vi "getData.vi"() -> (1 "Analogue Data (volts)":dbl[][](array[numeric]), 2 "Error Status":bool)   [LabVIEW 2017]
uses:
  Controls/blockTiming.ctl
  Globals/measurementGlobal.vi
panel:
  in  "display write dialog?":bool
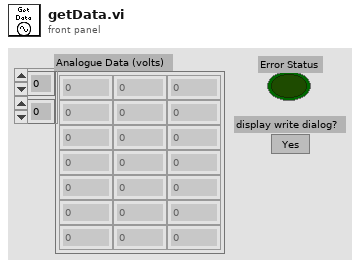
[diagram p1: front panel]
types:
  T1 = enum16{"New Measurement", "Post-process Raw Data"}
  T2 = typedef "blockTiming.ctl" = cluster{"Started":string, "Ended":string, "Analogue Frequency (Hz)":dbl}
  T3 = typedef "saveDataOption.ctl" = enum16{"Save Data", "Do Not Save Data"}
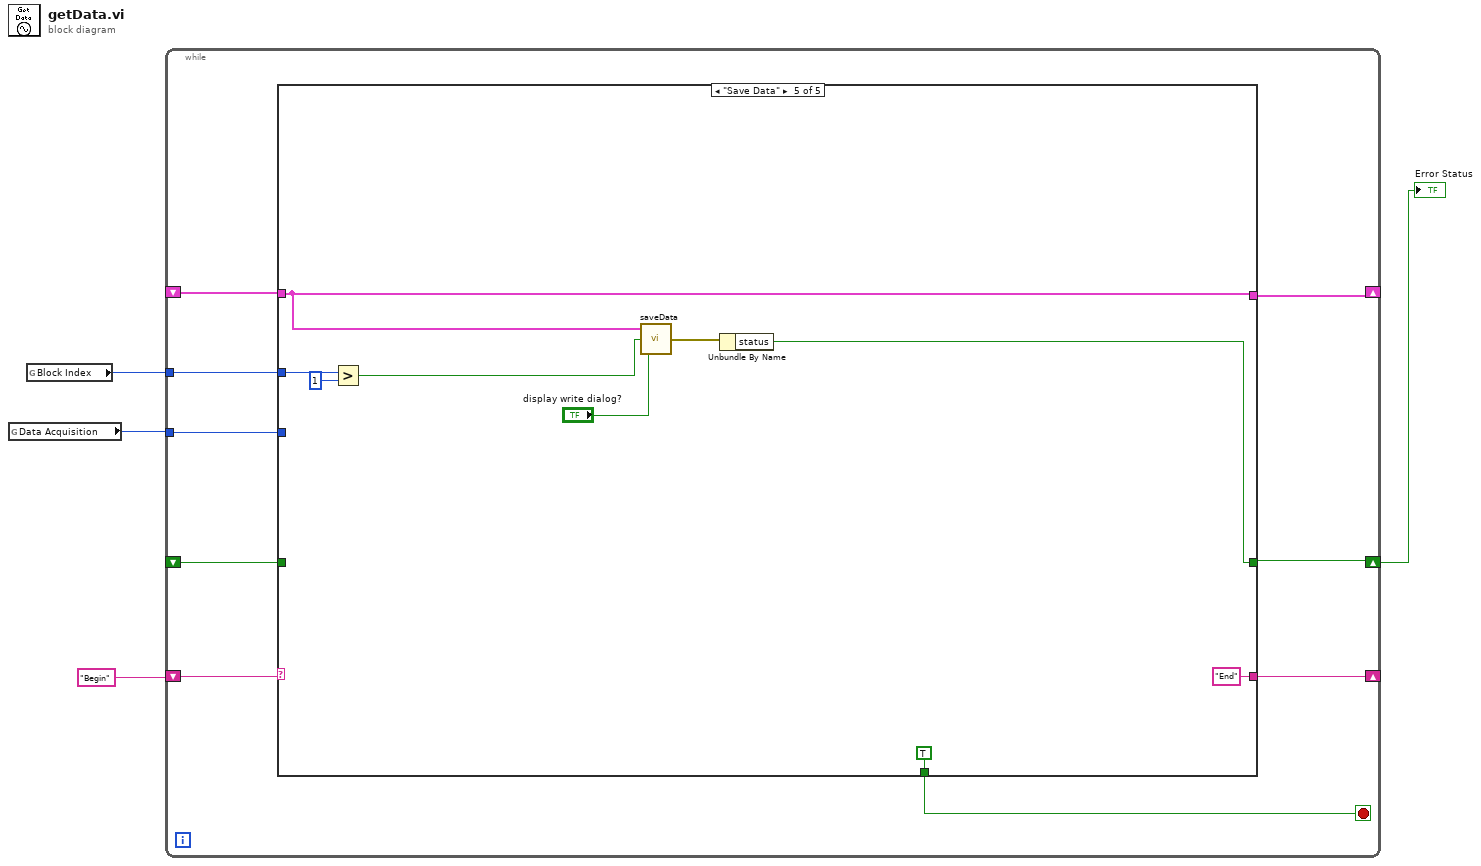
[diagram p0: block diagram]
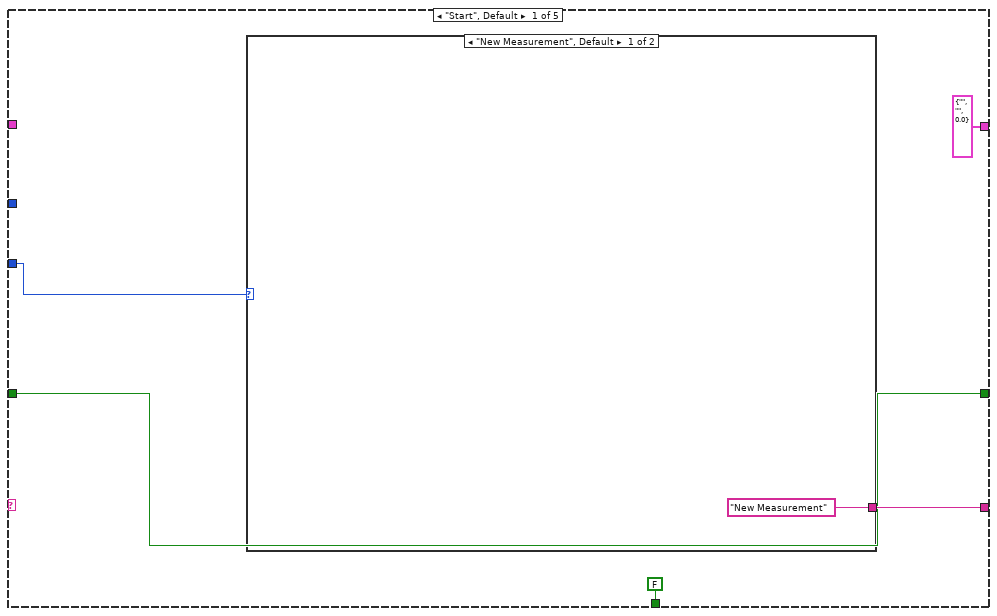
[diagram p2: hidden frame]
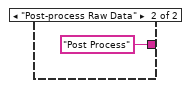
[diagram p3: hidden frame]
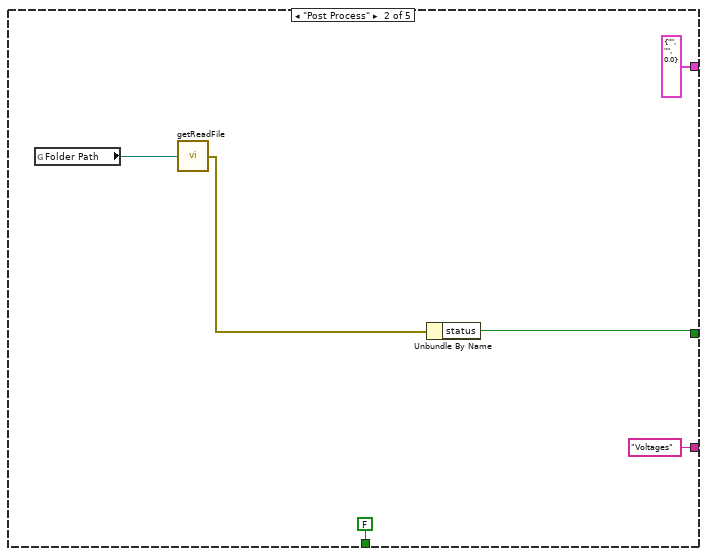
[diagram p4: hidden frame]
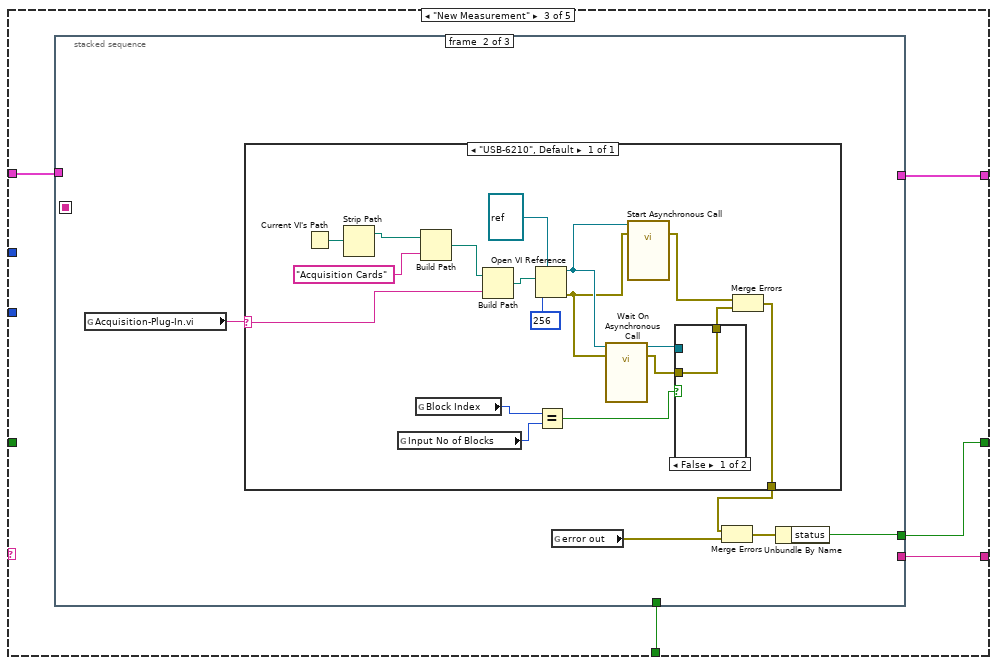
[diagram p5: hidden frame]
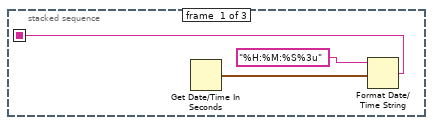
[diagram p6: hidden frame]
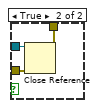
[diagram p7: hidden frame]
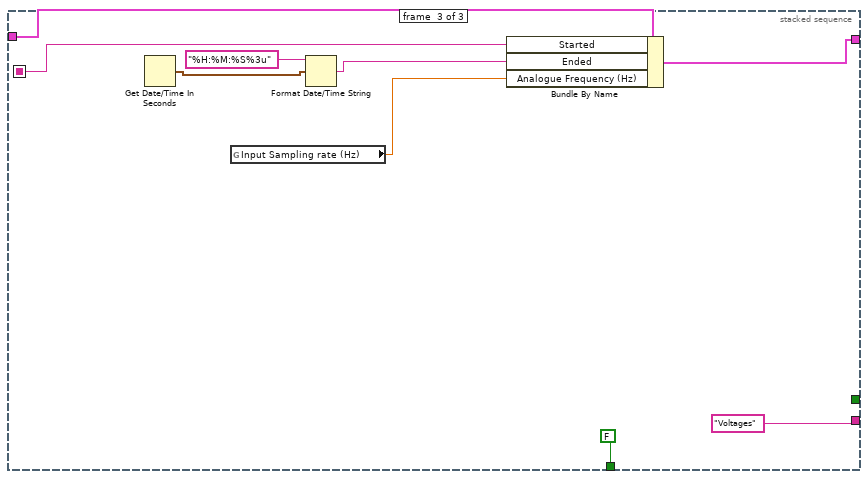
[diagram p8: hidden frame]
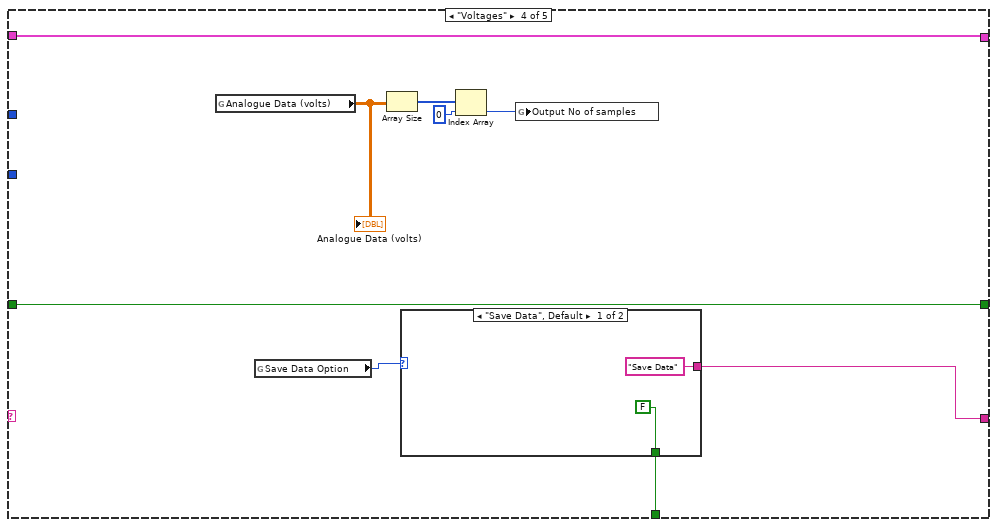
[diagram p9: hidden frame]
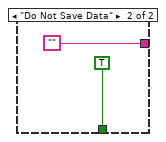
[diagram p10: hidden frame]
diagram:
  n1 = global read "measurementGlobal.vi" "Data Acquisition"() -> (w3:T1)
  n2 = global read "measurementGlobal.vi" "Block Index"() -> (w1:i32)
  n3 = while {
    tunnel: w3 -> [w12]
    shift-right: [w8] -> _
    shift-left: "Begin" -> [w13]
    shift-right: [w11] -> w2
    shift-left: _ -> [w9]
    shift-right: [w6] -> _
    shift-left: _ -> [w7]
    tunnel: w1 -> [w5]
    stop <- w10 stop-if-true
    n4 = case shown="\"Save Data\"" w13 {
      tunnel: w12 -> [w18 _ _ _ _]
      tunnel: [w17 "Voltages" w30 w72 "End"] -> w8
      tunnel: [w16 w25 w31 w74 w90] -> w11
      tunnel: [FALSE FALSE w29 w75 TRUE] -> w10
      tunnel: w9 -> [w16 _ _ w74 _]
      tunnel: w7 -> [_ _ w28 w73 w86]
      tunnel: [T2 {"Started"="", "Ended"="", "Analogue Frequency (Hz)"=0.0} ("Block Timing") T2 {"Started"="", "Ended"="", "Analogue Frequency (Hz)"=0.0} ("Block Timing") w27 w73 w86] -> w6
      tunnel: w5 -> [_ _ _ _ w92]
      frame "Start", Default {
        n5 = case shown="\"New Measurement\", Default" w18 {
          tunnel: ["New Measurement" "Post Process"] -> w17
          frame "New Measurement", Default {
          }
          frame "Post-process Raw Data" {
          }
        }
      }
      frame "Post Process" {
        n6 = global read "measurementGlobal.vi" "Folder Path"() -> (w21:path)
        n7 = call "getReadFile.vi"("Folder Path"=w21) -> ("error out"=w26:errorcluster)
        n8 = Unbundle By Name(w26) -> ("status"=w25:bool)
      }
      frame "New Measurement" {
        n9 = stacked-sequence {
          seq-local: [w33 _ _] -> [_ _ w68]
          tunnel: [_ w35 _] -> w31
          tunnel: [_ _ "Voltages"] -> w30
          tunnel: [_ _ FALSE] -> w29
          tunnel: w28 -> [_ _ w65]
          tunnel: [_ _ w66] -> w27
          frame #0 {
            n10 = Get Date/Time In Seconds() -> (seconds since 1Jan1904=w34:timestamp)
            n11 = Format Date/Time String(time format string (%c)="%H:%M:%S%3u", seconds (now)=w34) -> (date/time string=w33:string)  [unwired: 1 in]
          }
          frame #1 {
            n12 = global read "measurementGlobal.vi" "Acquisition-Plug-In.vi"() -> (w39:string)
            n13 = case shown="\"USB-6210\", Default" w39 {
              selector: w39 -> [w56]
              tunnel: [w54] -> w38
              frame "USB-6210", Default {
                n14 = Current VI's Path() -> (path=w57:path)
                n15 = Strip Path(path=w57) -> (stripped path=w46:path)  [unwired: 1 out]
                n16 = global read "measurementGlobal.vi" "Input No of Blocks"() -> (w50:i32)
                n17 = global read "measurementGlobal.vi" "Block Index"() -> (w51:i32)
                n18 = Build Path(base path=w46, name or relative path="Acquisition Cards") -> (appended path=w45:path)
                n19 = Build Path(base path=w45, name or relative path=w56) -> (appended path=w52:path)
                n20 = Open VI Reference(type specifier VI Refnum (for type only)=refnum<vi> refnum, vi path=w52, options=256) -> (vi reference=w42:refnum<vi>, error out=w41:errorcluster)  [unwired: 3 in]
                n21 = Equal?(x=w51, y=w50) -> (x = y?=w49:bool)
                n22 = call-by-ref "Wait On Asynchronous Call"(reference=w42, error in=w41) -> (reference out=w44:refnum<vi>, error out=w43:errorcluster)  [unwired: 1 in, 1 out]
                n23 = call-by-ref "Start Asynchronous Call"(reference=w42, error in=w41) -> (error out=w40:errorcluster)  [unwired: 1 in, 2 out]
                n24 = case shown="False" w49 {
                  tunnel: w44 -> [_ w61]
                  tunnel: w43 -> [w58 w60]
                  tunnel: [w58 w59] -> w55
                  frame False {
                  }
                  frame True {
                    n25 = Close Reference(reference=w61, error in (no error)=w60) -> (error out=w59:errorcluster)
                  }
                }
                n26 = Merge Errors(w40, w55) -> (w54:errorcluster)
              }
            }
            n27 = global read "measurementGlobal.vi" "error out"() -> (w37:errorcluster)
            n28 = Merge Errors(w38, w37) -> (w36:errorcluster)
            n29 = Unbundle By Name(w36) -> ("status"=w35:bool)
          }
          frame #2 {
            n30 = Get Date/Time In Seconds() -> (seconds since 1Jan1904=w63:timestamp)
            n31 = global read "measurementGlobal.vi" "Input Sampling rate (Hz)"() -> (w67:dbl)
            n32 = Format Date/Time String(time format string (%c)="%H:%M:%S%3u", seconds (now)=w63) -> (date/time string=w62:string)  [unwired: 1 in]
            n33 = Bundle By Name(cluster=w65, "Started"=w68, "Ended"=w62, "Analogue Frequency (Hz)"=w67) -> (w66:T2)
          }
        }
      }
      frame "Voltages" {
        n34 = global read "measurementGlobal.vi" "Analogue Data (volts)"() -> (w71:dbl[][])
        "Analogue Data (volts)" <- w71
        n35 = global read "measurementGlobal.vi" "Save Data Option"() -> (w76:T3)
        n36 = Array Size(array=w71) -> (size(s)=w79:i32[])
        n37 = case shown="\"Save Data\", Default" w76 {
          tunnel: [FALSE TRUE] -> w75
          tunnel: ["Save Data" ""] -> w72
          frame "Save Data", Default {
          }
          frame "Do Not Save Data" {
          }
        }
        n38 = Index Array(array=w79, index=0) -> (element=w77:i32)
        n39 = global write "measurementGlobal.vi" "Output No of samples"(w77) -> ()
      }
      frame "Save Data" {
        n40 = Greater?(x=w92, y=1) -> (0:w84:bool)
        n41 = call "saveData.vi"("display write dialog?"="display write dialog?", "append to file?"=w84, "Block Timing"=w86) -> ("error out"=w87:errorcluster)
        n42 = Unbundle By Name(w87) -> ("status"=w90:bool)
      }
    }
  }
  "Error Status" <- w2
